vi "TSM SSC Digital Write Static Per-Site.vi"(0 "Digital TSM In":T1, 5 "Per-Site State":T3[](array[typedef]) items=["0"=0, "1"=1, "X"=5], 11 "error in":errorcluster) -> (4 "Digital TSM Out":T1, 15 "error out":errorcluster)   [LabVIEW 2020]
doc: "Writes per-site static states to the specified pin(s) and pin group(s). The selected pins remain in the specified state until the next pattern burst or call to this VI. If there are uncommitted changes to levels or the termination mode, this VI commits the changes to the pins.\n\nThis VI does not change the selected pin function. If you write a static state to a pin that does not have the Digital function selected, the new static state is stored by the digital pattern instrument, and affects the state of the pin the next time you change the selected function to Digital."
uses:
  <instrlib>/niDigital/niDigital.llb/niDigital Write Static Pin State.ctl
  TSM/TSM SSC Digital.ctl
  <vilib>/NI_TestStand_SemiconductorModule/NI_TestStand_Semiconductor_Module.lvlibp/PinMap/Digital Pattern/PinQueryContext/DigitalPatternPinQueryContext.lvclass
  SSC Digital/SSC Digital.ctl
  15eee99f-1c92-4878-9705-bdf56774dbb6.vi
  Shared SubVIs/Site List to Site Numbers.vi
  Shared SubVIs/Channel List to Pins.vi
  Shared SubVIs/Trim Whitespace [Inlined].vi
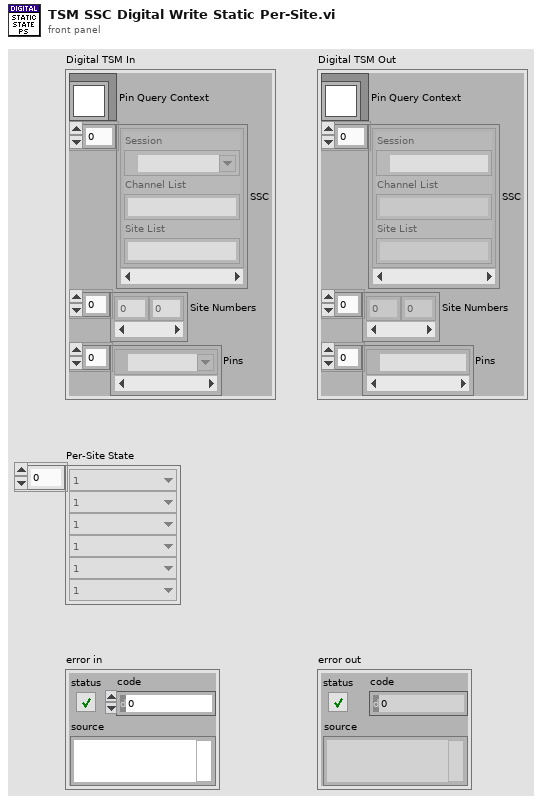
[diagram p1: front panel]
types:
  T1 = typedef "TSM SSC Digital.ctl" = cluster{"Pin Query Context":refnum<class "DigitalPatternPinQueryContext.lvclass">, "SSC":T2[], "Site Numbers":i32[], "Pins":tag[]}
  T2 = typedef "SSC Digital.ctl" = cluster{"Session":refnum<k15>, "Channel List":string, "Site List":string}
  T3 = typedef "niDigital Write Static Pin State.ctl" = u8
  T4 = typedef "Digital 2D Location.ctl" = cluster{"Row":i32, "Col":i32}
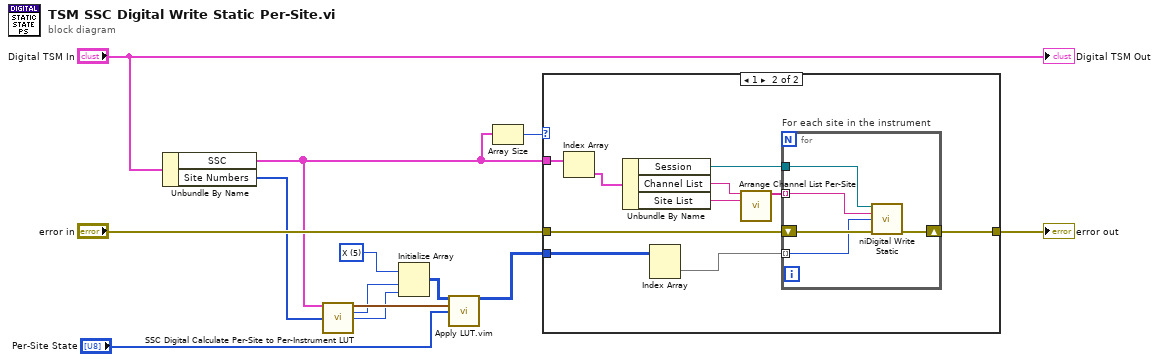
[diagram p0: block diagram]
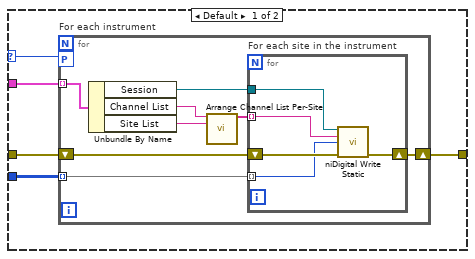
[diagram p2: hidden frame]
diagram:
  w5 = T3 5 items=["0"=0, "1"=1, "X"=5] ("State Per-Site")
  n1 = Unbundle By Name("Digital TSM In") -> ("SSC"=w1:T2[], "Site Numbers"=w6:i32[])
  n2 = call "SSC Digital Calculate Per-Site to Per-Instrument LUT.vi"("Digital SSC In"=w1, "Sites"=w6) -> ("Per-Site to Per-Instrument LUT"=w9:T4[], "Instrument Count"=w8:i32, "Max Sites on Instrument"=w7:i32)  [unwired: 11 in]
  n3 = Initialize Array(w5, w8, w7) -> (w10:T3[][])
  n4 = call "Apply LUT.vim"("Initialized Array"=w10, "LUT"=w9, "Results to Apply LUT to"="Per-Site State") -> ("Array Out"=w3:T3[][])  [unwired: 12 in]
  n5 = Array Size(array=w1) -> (size(s)=w2:i32)
  n6 = case shown="1" w2 {
    selector: w2 -> [w15 _]
    tunnel: [w18 w41] -> w13
    tunnel: "error in" -> [w17 w40]
    tunnel: w3 -> [w16 w39]
    tunnel: w1 -> [w14 w38]
    frame Default {
      n7 = for "For each instrument" {
        workers-P: w15 -> [_]
        tunnel: w14 -> [w24] mode=indexing
        shift-right: [w26] -> w18
        shift-left: w17 -> [w22]
        tunnel: w16 -> [w19] mode=indexing
        n8 = Unbundle By Name(w24) -> ("Session"=w23:refnum<k15>, "Channel List"=w21:string, "Site List"=w20:string)
        n9 = call "Arrange Channel List Per-Site.vi"("Channel List String"=w21, "Site List String"=w20) -> ("Channel List Array"=w25:string[])  [unwired: 11 in, 2 out]
        n10 = for "For each site in the instrument" {
          shift-right: [w30] -> w26
          shift-left: w22 -> [w31]
          tunnel: w25 -> [w29] mode=indexing
          tunnel: w23 -> [w28]
          tunnel: w19 -> [w27] mode=indexing
          n11 = call <instrlib>:"niDigital Write Static.vi"("instrument handle"=w28, "channel list"=w29, "state"=w27, "error in"=w31) -> ("error out"=w30:errorcluster)  [unwired: 10 in, 1 out]
        }
      }
    }
    frame 1 {
      n12 = Index Array(array=w38) -> (element=w33:T2)  [unwired: 1 in]
      n13 = Unbundle By Name(w33) -> ("Session"=w36:refnum<k15>, "Channel List"=w35:string, "Site List"=w34:string)
      n14 = Index Array(array=w39) -> (element=w32:T3[])  [unwired: 2 in]
      n15 = call "Arrange Channel List Per-Site.vi"("Channel List String"=w35, "Site List String"=w34) -> ("Channel List Array"=w37:string[])  [unwired: 11 in, 2 out]
      n16 = for "For each site in the instrument" {
        shift-right: [w45] -> w41
        shift-left: w40 -> [w46]
        tunnel: w37 -> [w44] mode=indexing
        tunnel: w36 -> [w43]
        tunnel: w32 -> [w42] mode=indexing
        n17 = call <instrlib>:"niDigital Write Static.vi"("instrument handle"=w43, "channel list"=w44, "state"=w42, "error in"=w46) -> ("error out"=w45:errorcluster)  [unwired: 10 in, 1 out]
      }
    }
  }
  "error out" <- w13
  "Digital TSM Out" <- "Digital TSM In"
